vi "Wärmepumpe.Heizleistung.vi"(8 "Error in":errorcluster, 9 "Rücklauftemperatur Solekreislauf [°C]":dbl, 10 "Rücklauftemperatur Heizkreislauf [°C]":dbl, 11 "Wärmepumpe in":refnum<data-value>) -> (0 "Error out":errorcluster, 3 "Wärmepumpe out":refnum<data-value>)   [LabVIEW 2016, in "Wärmepumpe.lvclass"]
uses:
  <vilib>/gmath/interp.llb/Interpolate 2D (1d xi,yi).vi
  <vilib>/gmath/NI_Gmath.lvlib
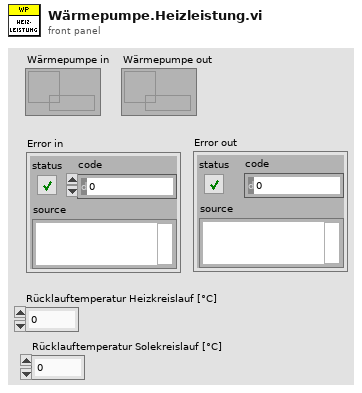
[diagram p1: front panel]
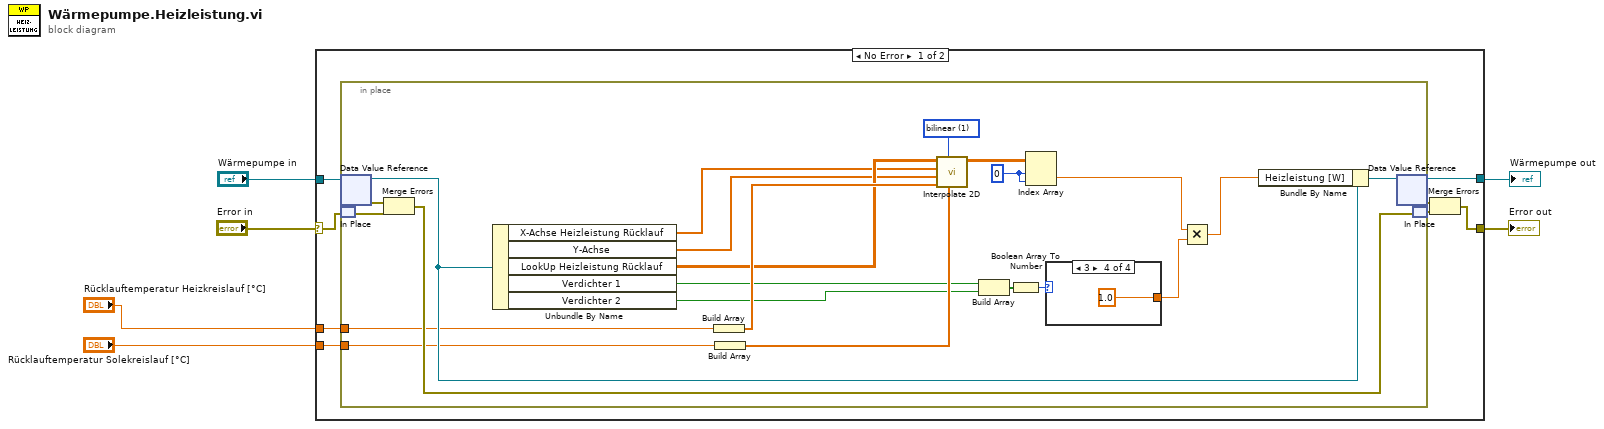
[diagram p0: block diagram]
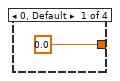
[diagram p2: hidden frame]
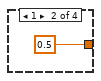
[diagram p3: hidden frame]
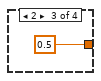
[diagram p4: hidden frame]
diagram:
  n1 = case shown="No Error" "Error in" {
    selector: "Error in" -> [w12 w42]
    tunnel: [w11 w41] -> w4
    tunnel: [w10 w42] -> w3
    tunnel: "Wärmepumpe in" -> [w9 w41]
    tunnel: "Rücklauftemperatur Heizkreislauf [°C]" -> [w8 _]
    tunnel: "Rücklauftemperatur Solekreislauf [°C]" -> [w7 _]
    frame No Error {
      n2 = in-place {
        in-place-border: w8 -> [w23]
        in-place-border: w7 -> [w22]
        w31 = 0 ("index (row)")
        w30 = 1 items=["nearest", "bilinear", "bicubic", "bicubic spline"] ("method")
        n3 = in-place-dvr #1(w9) -> (w29:refnum<class "Wärmepumpe.lvclass">, w36:errorcluster)
        n4 = in-place-match #2(w12) -> (w35:errorcluster)
        n5 = Merge Errors(w36, w35) -> (w34:errorcluster)
        n6 = Unbundle By Name(w29) -> ("X-Achse Heizleistung Rücklauf"=w25:dbl[], "Y-Achse"=w24:dbl[], "LookUp Heizleistung Rücklauf"=w26:dbl[][], "Verdichter 1"=w18:bool, "Verdichter 2"=w17:bool)
        n7 = Build Array(w23) -> (w28:dbl[])
        n8 = Build Array(w22) -> (w27:dbl[])
        n9 = call-poly <vilib>:"Interpolate 2D.vi"("yi"=w27, "method"=w30, "xi"=w28, "Y"=w24, "X"=w25, "Z"=w26) -> ("zi"=w32:dbl[][])  [unwired: 2 in, 3 out]
        n10 = Build Array(w18, w17) -> (w21:bool[])
        n11 = Boolean Array To Number(Boolean array=w21) -> (number=w20:u32)
        n12 = Index Array(array=w32, index (row)=w31, index (col)=w31) -> (element=w16:dbl)
        n13 = case shown="3" w20 {
          tunnel: [0.0 0.5 0.5 1.0] -> w19
          frame 0, Default {
          }
          frame 1 {
          }
          frame 2 {
          }
          frame 3 {
          }
        }
        n14 = Multiply(x=w16, y=w19) -> (x*y=w15:dbl)
        n15 = Bundle By Name(cluster=w29, "Heizleistung [W]"=w15) -> (w33:refnum<class "Wärmepumpe.lvclass">)
        n16 = in-place-dvr #1(w33) -> (w11:refnum<data-value>, w14:errorcluster)
        n17 = in-place-match #2(w34) -> (w13:errorcluster)
      }
      n18 = Merge Errors(w14, w13) -> (w10:errorcluster)
    }
    frame Error {
    }
  }
  "Wärmepumpe out" <- w4
  "Error out" <- w3
